vi "getEndTone.vi"(8 "error in (no error)":errorcluster, 11 "RampTone.lvclass in":refnum<class "RampTone.lvclass">) -> (0 "error out":errorcluster, 2 "endTone.lvclass":refnum<class "SingleTone.lvclass">, 3 "RampTone.lvclass out":refnum<class "RampTone.lvclass">)   [LabVIEW 2009, in "Tools.lvlib" / "Scripting.lvlib" / "RampTone.lvclass"]
uses:
  RampTone.lvclass
  SingleTone/SingleTone.lvclass
  RampTone.lvclass/RampTone.ctl
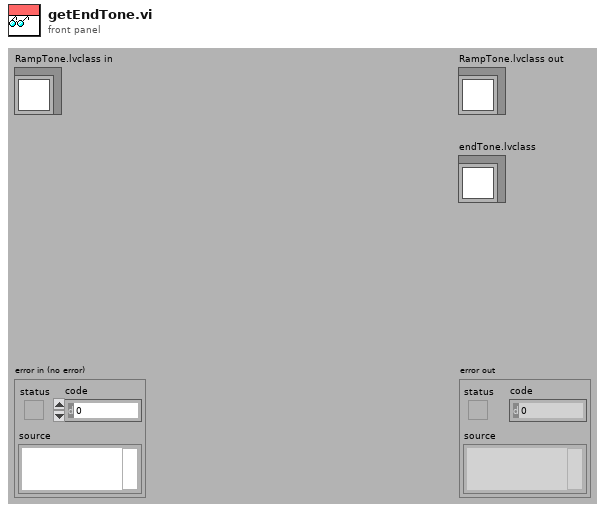
[diagram p1: front panel]
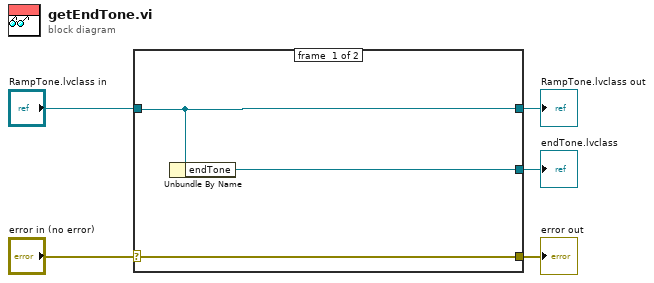
[diagram p0: block diagram]
diagram:
  n1 = case shown="No Error" "error in (no error)" {
    selector: "error in (no error)" -> [w8 w9]
    tunnel: [w8 w9] -> w4
    tunnel: [w7 w10] -> w2
    tunnel: "RampTone.lvclass in" -> [w7 w10]
    tunnel: [w6 _] -> w1
    frame #0 {
      n2 = Unbundle By Name(w7) -> ("endTone"=w6:refnum<class "SingleTone.lvclass">)
    }
    frame #1 {
    }
  }
  "error out" <- w4
  "RampTone.lvclass out" <- w2
  "endTone.lvclass" <- w1
